vi "Filterwheel.vi"(5 "network settings":T2, 7 "Mode":u16(ring)=1 items=["Init", "Update"], 8 "error in":errorcluster, 10 "Filters&shutters old value":T1={"vis+ND3"=FALSE, "IR+ND2"=FALSE, "Shutter Filterwheel"=TRUE, "Lambda Filterwheel 2"=1, "ND filterwheel 2"=1, "Epi Shutter 2"=FALSE} {"ND filterwheel 2" items=["ND0"=4, "ND1"=6, "ND2"=1, "ND3"=3, "ND4"=2]; "Lambda Filterwheel 2" items=["IR"=1, ""=2, "E440sp"=6]}, 11 "Filters&shutters":T1 {"ND filterwheel 2" items=["ND10"=1, "ND20"=2, "ND30"=3, "ND40"=4, "ND INFINITY"=5, "ND0"=6]; "Lambda Filterwheel 2" items=["IR"=1, "ND50"=2, "ND0"=3, "Green"=4, "Blue"=5, "ND0"=6]}) -> (0 "error out":errorcluster, 2 "String description":string, 3 "Filters&shutters Out":T1 {"ND filterwheel 2" items=["ND10"=1, "ND20"=2, "ND30"=3, "ND40"=4, "ND INFINITY"=5, "ND0"=6]; "Lambda Filterwheel 2" items=["IR"=1, "ND50"=2, "ND0"=3, "Green"=4, "Blue"=5, "ND0"=6]}, 4 "ND FW Strings And Values []":cluster{"String":string, "Value":u16}[](array[cluster]), 6 "Lambda FW Strings And Values []":cluster{"String":string, "Value":u16}[](array[cluster]))   [LabVIEW 2009]
panel:
  in  "Case Constant\n(See Context Help) 4":bool
  in  "Case Constant\n(See Context Help) 3":bool
  in  "Case Constant\n(See Context Help) 2":bool
  in  "Case Constant\n(See Context Help)":bool
  out "Lambda Filterwheel 2":u16(ring)=2 items=["IR"=1, ""=2, "E440sp"=6]
  out "ND filterwheel 2":u16(ring)=1 items=["ND0"=4, "ND1"=6, "ND2"=1, "ND3"=3, "ND4"=2]
  out "EpiShutter":bool
  out "Shutter Filterwheel":bool caption="Filterwheel"
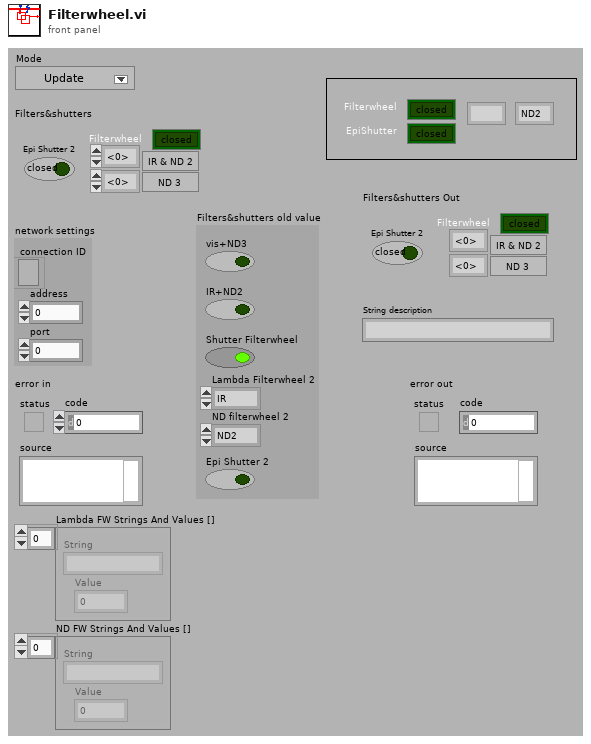
[diagram p1: front panel]
types:
  T1 = cluster{"vis+ND3":bool, "IR+ND2":bool, "Shutter Filterwheel":bool, "Lambda Filterwheel 2":u16, "ND filterwheel 2":u16, "Epi Shutter 2":bool}
  T2 = cluster{"connection ID":refnum<k16>, "address":u32, "port":u16}
  T3 = typedef "LVStringsAndValuesArrayTypeDef.ctl" = cluster{"String":string, "Value":u16}[]
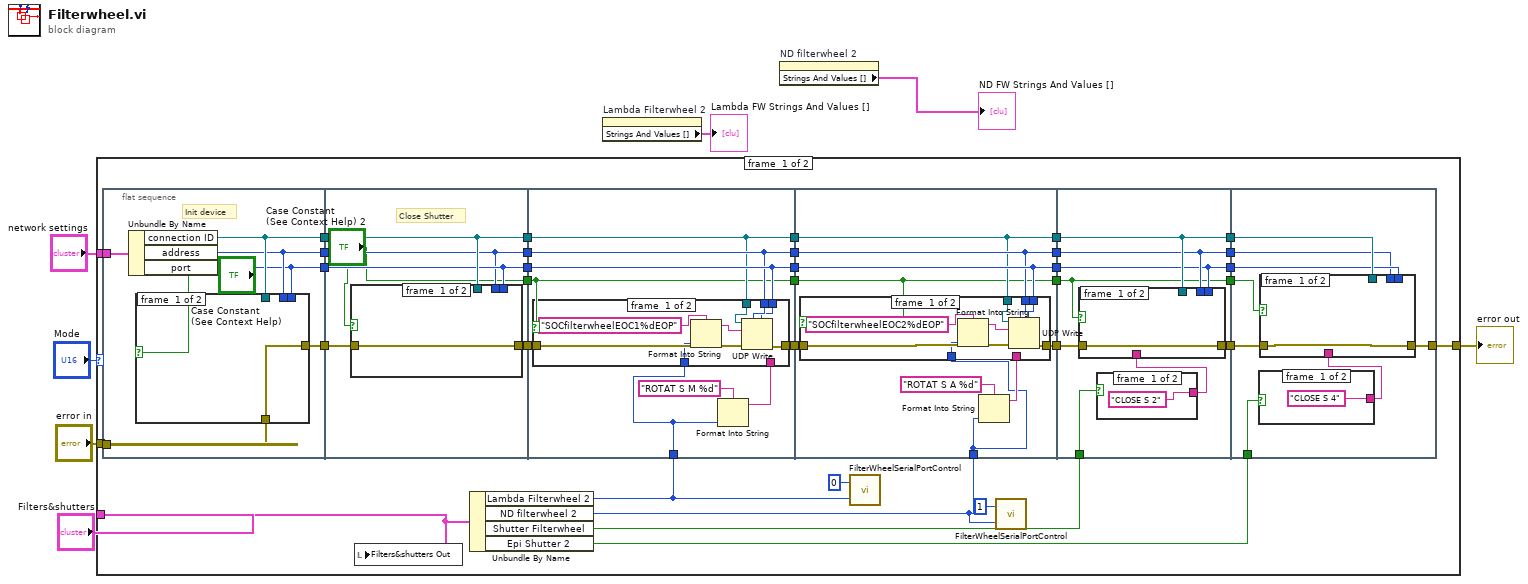
[diagram p0: block diagram]
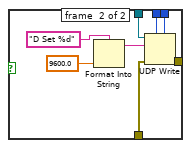
[diagram p2: hidden frame]
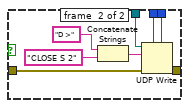
[diagram p3: hidden frame]
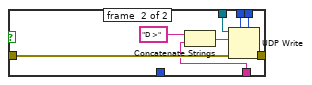
[diagram p4: hidden frame]
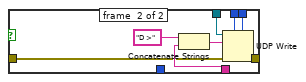
[diagram p5: hidden frame]
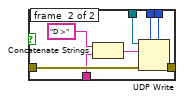
[diagram p6: hidden frame]
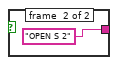
[diagram p7: hidden frame]
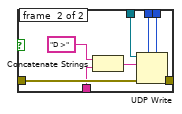
[diagram p8: hidden frame]
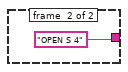
[diagram p9: hidden frame]
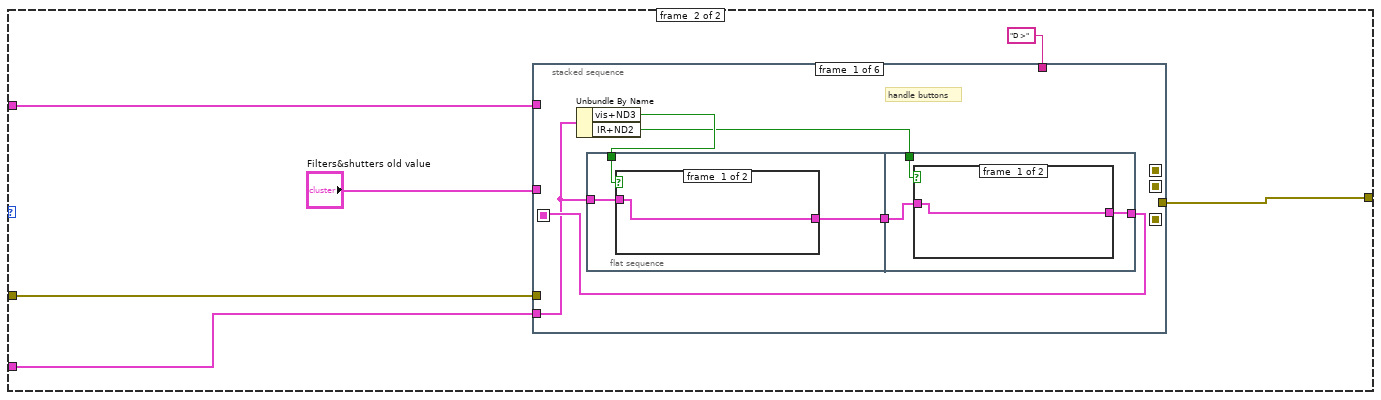
[diagram p10: hidden frame]
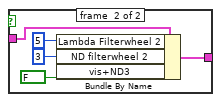
[diagram p11: hidden frame]
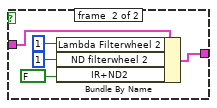
[diagram p12: hidden frame]
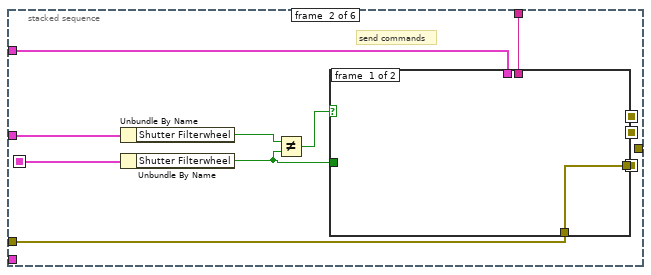
[diagram p13: hidden frame]
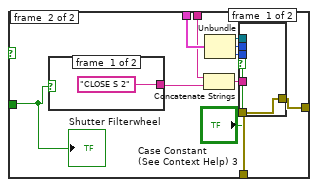
[diagram p14: hidden frame]
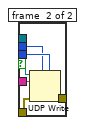
[diagram p15: hidden frame]
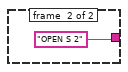
[diagram p16: hidden frame]
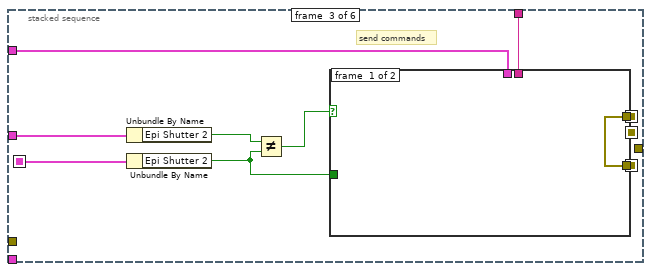
[diagram p17: hidden frame]
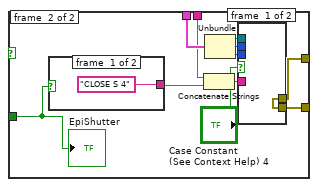
[diagram p18: hidden frame]
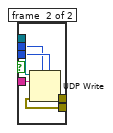
[diagram p19: hidden frame]
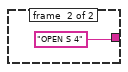
[diagram p20: hidden frame]
diagram:
  n1 = case shown="1, Default" "Mode" {
    tunnel: "network settings" -> [w41 w164]
    tunnel: "error in" -> [w40 w163]
    tunnel: [w39 w162] -> w4
    tunnel: "Filters&shutters" -> [w21 w161]
    frame #0 {
      n2 = flat-sequence {
        tunnel: w41 -> [w48]
        tunnel: w40 -> [w47]
        tunnel: [w46] -> w38
        tunnel: [w45] -> w37
        tunnel: [w44] -> w36
        tunnel: [w43] -> w35
        tunnel: w38 -> [w63]
        tunnel: w37 -> [w61]
        tunnel: w36 -> [w59]
        tunnel: w35 -> [w60]
        tunnel: [w62] -> w34
        tunnel: [w61] -> w33
        tunnel: [w60] -> w32
        tunnel: [w59] -> w31
        tunnel: ["Case Constant\n(See Context Help) 2"] -> w11
        tunnel: w34 -> [w81]
        tunnel: w33 -> [w77]
        tunnel: [w77] -> w29
        tunnel: w32 -> [w79]
        tunnel: [w79] -> w27
        tunnel: w31 -> [w78]
        tunnel: [w78] -> w25
        tunnel: [w80] -> w30
        tunnel: w15 -> [w73]
        tunnel: w11 -> [w74]
        tunnel: [w74] -> w10
        tunnel: w30 -> [w103]
        tunnel: w29 -> [w100]
        tunnel: [w100] -> w28
        tunnel: w27 -> [w102]
        tunnel: [w102] -> w26
        tunnel: w25 -> [w101]
        tunnel: [w101] -> w24
        tunnel: [w104] -> w23
        tunnel: w14 -> [w98]
        tunnel: w10 -> [w99]
        tunnel: [w99] -> w9
        tunnel: w23 -> [w130]
        tunnel: w28 -> [w126]
        tunnel: w26 -> [w124]
        tunnel: w24 -> [w125]
        tunnel: w22 -> [w127]
        tunnel: [w129] -> w20
        tunnel: [w126] -> w19
        tunnel: [w125] -> w18
        tunnel: [w124] -> w17
        tunnel: w9 -> [w123]
        tunnel: [w123] -> w8
        tunnel: [w148] -> w39
        tunnel: w20 -> [w149]
        tunnel: w19 -> [w147]
        tunnel: w18 -> [w145]
        tunnel: w17 -> [w146]
        tunnel: w16 -> [w143]
        tunnel: w8 -> [w142]
        frame #0 {
          # "Init device"
          n3 = Unbundle By Name(w48) -> ("connection ID"=w45:refnum<k16>, "address"=w44:u32, "port"=w43:u16)
          n4 = case shown="True" "Case Constant\n(See Context Help)" {
            tunnel: w47 -> [w49 w54]
            tunnel: [w49 w53] -> w46
            tunnel: w45 -> [_ w52]
            tunnel: w44 -> [_ w51]
            tunnel: w43 -> [_ w50]
            frame #0 {
            }
            frame #1 {
              n5 = Format Into String(format string="D Set %d", 9600.0 ("input 1")) -> (resulting string=w57:string)  [unwired: 2 in, 1 out]
              n6 = UDP Write(address=w51, port or service name=w50, connection ID=w52, data in=w57, 8:w54) -> (error out=w53:errorcluster)  [unwired: 1 in, 1 out]
            }
          }
        }
        frame #1 {
          # "Close Shutter"
          n7 = case shown="True" "Case Constant\n(See Context Help) 2" {
            tunnel: w63 -> [w64 w69]
            tunnel: [w64 w68] -> w62
            tunnel: w61 -> [_ w67]
            tunnel: w60 -> [_ w66]
            tunnel: w59 -> [_ w65]
            frame #0 {
            }
            frame #1 {
              n8 = Concatenate Strings("D >" ("string"), "CLOSE S 2") -> (w70:string)
              n9 = UDP Write(address=w65, port or service name=w66, connection ID=w67, data in=w70, 8:w69) -> (error out=w68:errorcluster)  [unwired: 1 in, 1 out]
            }
          }
        }
        frame #2 {
          n10 = Format Into String(format string="ROTAT S M %d", w73) -> (resulting string=w75:string)  [unwired: 2 in, 1 out]
          n11 = case shown="True" w74 {
            tunnel: w81 -> [w86 w95]
            tunnel: [w85 w94] -> w80
            tunnel: w79 -> [w88 w93]
            tunnel: w78 -> [w89 w92]
            tunnel: w77 -> [w87 w91]
            tunnel: w75 -> [_ w90]
            tunnel: w73 -> [w83 _]
            frame #0 {
              n12 = Format Into String(format string="SOCfilterwheelEOC1%dEOP" ("initial string"), w83) -> (resulting string=w84:string)  [unwired: 2 in, 1 out]
              n13 = UDP Write(address=w89, port or service name=w88, connection ID=w87, data in=w84, 8:w86) -> (error out=w85:errorcluster)  [unwired: 1 in, 1 out]
            }
            frame #1 {
              n14 = Concatenate Strings("D >" ("string"), w90) -> (w96:string)
              n15 = UDP Write(address=w92, port or service name=w93, connection ID=w91, data in=w96, 8:w95) -> (error out=w94:errorcluster)  [unwired: 1 in, 1 out]
            }
          }
        }
        frame #3 {
          n16 = Format Into String(format string="ROTAT S A %d", w98) -> (resulting string=w106:string)  [unwired: 2 in, 1 out]
          n17 = case shown="True" w99 {
            tunnel: w106 -> [_ w122]
            tunnel: [w112 w119] -> w104
            tunnel: w103 -> [w113 w118]
            tunnel: w102 -> [w108 w117]
            tunnel: w101 -> [w109 w116]
            tunnel: w100 -> [w110 w115]
            tunnel: w98 -> [w111 _]
            frame #0 {
              n18 = Format Into String(format string="SOCfilterwheelEOC2%dEOP" ("initial string"), w111) -> (resulting string=w114:string)  [unwired: 2 in, 1 out]
              n19 = UDP Write(address=w109, port or service name=w108, connection ID=w110, data in=w114, 8:w113) -> (error out=w112:errorcluster)  [unwired: 1 in, 1 out]
            }
            frame #1 {
              n20 = Concatenate Strings("D >" ("string"), w122) -> (w121:string)
              n21 = UDP Write(address=w116, port or service name=w117, connection ID=w115, data in=w121, 8:w118) -> (error out=w119:errorcluster)  [unwired: 1 in, 1 out]
            }
          }
        }
        frame #4 {
          n22 = case shown="True" w127 {
            tunnel: ["CLOSE S 2" "OPEN S 2"] -> w128
            frame #0 {
            }
            frame #1 {
            }
          }
          n23 = case shown="True" w123 {
            tunnel: w130 -> [w131 w137]
            tunnel: [w131 w136] -> w129
            tunnel: w128 -> [_ w135]
            tunnel: w126 -> [_ w134]
            tunnel: w125 -> [_ w133]
            tunnel: w124 -> [_ w132]
            frame #0 {
            }
            frame #1 {
              n24 = Concatenate Strings("D >" ("string"), w135) -> (w139:string)
              n25 = UDP Write(address=w133, port or service name=w132, connection ID=w134, data in=w139, 8:w137) -> (error out=w136:errorcluster)  [unwired: 1 in, 1 out]
            }
          }
        }
        frame #5 {
          n26 = case shown="True" w143 {
            tunnel: ["CLOSE S 4" "OPEN S 4"] -> w144
            frame #0 {
            }
            frame #1 {
            }
          }
          n27 = case shown="True" w142 {
            tunnel: w149 -> [w150 w156]
            tunnel: [w150 w155] -> w148
            tunnel: w147 -> [_ w154]
            tunnel: w146 -> [_ w153]
            tunnel: w145 -> [_ w152]
            tunnel: w144 -> [_ w151]
            frame #0 {
            }
            frame #1 {
              n28 = Concatenate Strings("D >" ("string"), w151) -> (w157:string)
              n29 = UDP Write(address=w152, port or service name=w153, connection ID=w154, data in=w157, 8:w156) -> (error out=w155:errorcluster)  [unwired: 1 in, 1 out]
            }
          }
        }
      }
      n30 = local write "Filters&shutters Out"(w21) -> ()
      n31 = Unbundle By Name(w21) -> ("Lambda Filterwheel 2"=w15:u16, "ND filterwheel 2"=w14:u16, "Shutter Filterwheel"=w22:bool, "Epi Shutter 2"=w16:bool)
      n32 = call "FilterWheelSerialPortControl.vi"("position"=w15, "channel"=u8 0) -> ()  [unwired: 1 out]
      n33 = call "FilterWheelSerialPortControl.vi"("position"=w14, "channel"=u8 1) -> ()  [unwired: 1 out]
    }
    frame #1 {
      n34 = stacked-sequence {
        seq-local: [_ w195 _ _ _ _] -> [_ _ w225 _ _ _]
        seq-local: [_ _ w224 _ _ _] -> [_ _ _ w254 w275 _]
        seq-local: [_ _ _ _ w274 _] -> [_ _ _ _ _ w294]
        seq-local: [w168 _ _ _ _ _] -> [_ w192 w221 w251 w271 w293]
        tunnel: w164 -> [_ w198 w228 w257 w278 _]
        tunnel: "D >" ("string") -> [_ w197 w227 w256 w277 _]
        tunnel: w163 -> [_ w190 _ _ _ _]
        tunnel: [_ _ _ _ _ w294] -> w162
        tunnel: "Filters&shutters old value" -> [_ w194 w223 w253 w273 _]
        tunnel: w161 -> [w167 _ _ _ _ _]
        frame #0 {
          # "handle buttons"
          n35 = Unbundle By Name(w167) -> ("vis+ND3"=w170:bool, "IR+ND2"=w169:bool)
          n36 = flat-sequence {
            tunnel: w167 -> [w174]
            tunnel: [w173] -> w171
            tunnel: w170 -> [w172]
            tunnel: w171 -> [w183]
            tunnel: w169 -> [w182]
            tunnel: [w181] -> w168
            frame #0 {
              n37 = case shown="True" w172 {
                tunnel: w174 -> [w175 w180]
                tunnel: [w175 w176] -> w173
                frame #0 {
                }
                frame #1 {
                  n38 = Bundle By Name(cluster=w180, "Lambda Filterwheel 2"=u16 5, "ND filterwheel 2"=u16 3, "vis+ND3"=FALSE) -> (w176:T1)
                }
              }
            }
            frame #1 {
              n39 = case shown="True" w182 {
                tunnel: w183 -> [w184 w189]
                tunnel: [w184 w185] -> w181
                frame #0 {
                }
                frame #1 {
                  n40 = Bundle By Name(cluster=w189, "Lambda Filterwheel 2"=u16 1, "ND filterwheel 2"=u16 1, "IR+ND2"=FALSE) -> (w185:T1)
                }
              }
            }
          }
        }
        frame #1 {
          # "send commands"
          n41 = Unbundle By Name(w194) -> ("Shutter Filterwheel"=w193:bool)
          n42 = Unbundle By Name(w192) -> ("Shutter Filterwheel"=w191:bool)
          n43 = Not Equal?(x=w193, y=w191) -> (x != y?=w196:bool)
          n44 = case shown="True" w196 {
            tunnel: w198 -> [_ w205]
            tunnel: w197 -> [_ w204]
            tunnel: w190 -> [w199 w203]
            tunnel: [w199 w202] -> w195
            tunnel: w191 -> [_ w201]
            frame #0 {
            }
            frame #1 {
              n45 = case shown="False" w201 {
                tunnel: ["CLOSE S 2" "OPEN S 2"] -> w206
                frame #0 {
                }
                frame #1 {
                }
              }
              n46 = Concatenate Strings(w204, w206) -> (w210:string)
              n47 = Unbundle(w205) -> ("connection ID"=w209:refnum<k16>, "address"=w207:u32, "port"=w208:u16)
              n48 = case shown="True" "Case Constant\n(See Context Help) 3" {
                tunnel: w210 -> [_ w217]
                tunnel: w209 -> [_ w216]
                tunnel: w208 -> [_ w215]
                tunnel: w207 -> [_ w214]
                tunnel: w203 -> [w211 w213]
                tunnel: [w211 w212] -> w202
                frame #0 {
                }
                frame #1 {
                  n49 = UDP Write(address=w214, port or service name=w215, connection ID=w216, data in=w217, 8:w213) -> (error out=w212:errorcluster)  [unwired: 1 in, 1 out]
                }
              }
              "Shutter Filterwheel" <- w201
            }
          }
        }
        frame #2 {
          # "send commands"
          n50 = Unbundle By Name(w223) -> ("Epi Shutter 2"=w222:bool)
          n51 = Unbundle By Name(w221) -> ("Epi Shutter 2"=w220:bool)
          n52 = Not Equal?(x=w222, y=w220) -> (x != y?=w226:bool)
          n53 = case shown="True" w226 {
            tunnel: w228 -> [_ w235]
            tunnel: w227 -> [_ w234]
            tunnel: w225 -> [w229 w233]
            tunnel: [w229 w232] -> w224
            tunnel: w220 -> [_ w231]
            frame #0 {
            }
            frame #1 {
              n54 = case shown="True" w231 {
                tunnel: ["CLOSE S 4" "OPEN S 4"] -> w236
                frame #0 {
                }
                frame #1 {
                }
              }
              n55 = Concatenate Strings(w234, w236) -> (w240:string)
              n56 = Unbundle(w235) -> ("connection ID"=w239:refnum<k16>, "address"=w237:u32, "port"=w238:u16)
              n57 = case shown="True" "Case Constant\n(See Context Help) 4" {
                tunnel: w240 -> [_ w247]
                tunnel: w239 -> [_ w246]
                tunnel: w238 -> [_ w245]
                tunnel: w237 -> [_ w244]
                tunnel: w233 -> [w241 w243]
                tunnel: [w241 w242] -> w232
                frame #0 {
                }
                frame #1 {
                  n58 = UDP Write(address=w244, port or service name=w245, connection ID=w246, data in=w247, 8:w243) -> (error out=w242:errorcluster)  [unwired: 1 in, 1 out]
                }
              }
              "EpiShutter" <- w231
            }
          }
        }
        frame #3 {
          # "send commands"
          n59 = Unbundle By Name(w253) -> ("Lambda Filterwheel 2"=w252:u16)
          n60 = Unbundle By Name(w251) -> ("Lambda Filterwheel 2"=w250:u16)
          n61 = Not Equal?(x=w252, y=w250) -> (x != y?=w255:bool)
          n62 = case shown="True" w255 {
            tunnel: w257 -> [_ w266]
            tunnel: w256 -> [_ w265]
            tunnel: w254 -> [_ w262]
            tunnel: w250 -> [_ w260]
            frame #0 {
            }
            frame #1 {
              n63 = call "FilterWheelSerialPortControl.vi"("position"=w260, "channel"=u8 0) -> ()  [unwired: 1 out]
              n64 = Format Into String(format string="ROTAT S M %d", w260) -> (resulting string=w263:string)  [unwired: 2 in, 1 out]
              n65 = Unbundle(w266) -> ("connection ID"=w269:refnum<k16>, "address"=w267:u32, "port"=w268:u16)
              n66 = Concatenate Strings(w265, w263) -> ()  [unwired: 1 out]
              n67 = Format Into String(format string="SOCfilterwheelEOC0,%dEOP" ("initial string"), w260) -> (resulting string=w259:string)  [unwired: 2 in, 1 out]
              n68 = UDP Write(address=w267, port or service name=w268, connection ID=w269, data in=w259, 8:w262) -> ()  [unwired: 1 in, 2 out]
              "Lambda Filterwheel 2" <- w260
            }
          }
        }
        frame #4 {
          # "send commands"
          n69 = Unbundle By Name(w273) -> ("ND filterwheel 2"=w272:u16)
          n70 = Unbundle By Name(w271) -> ("ND filterwheel 2"=w270:u16)
          n71 = Not Equal?(x=w272, y=w270) -> (x != y?=w276:bool)
          n72 = case shown="True" w276 {
            tunnel: w278 -> [_ w289]
            tunnel: w277 -> [_ w288]
            tunnel: w275 -> [w279 w285]
            tunnel: [w279 w284] -> w274
            tunnel: w270 -> [_ w282]
            frame #0 {
            }
            frame #1 {
              n73 = call "FilterWheelSerialPortControl.vi"("position"=w282, "channel"=u8 1) -> ()  [unwired: 1 out]
              n74 = Format Into String(format string="ROTAT S A %d", w282) -> (resulting string=w286:string)  [unwired: 2 in, 1 out]
              n75 = Unbundle(w289) -> ("connection ID"=w292:refnum<k16>, "address"=w290:u32, "port"=w291:u16)
              n76 = Concatenate Strings(w288, w286) -> ()  [unwired: 1 out]
              n77 = Format Into String(format string="SOCfilterwheelEOC1,%dEOP" ("initial string"), w282) -> (resulting string=w281:string)  [unwired: 2 in, 1 out]
              n78 = UDP Write(address=w290, port or service name=w291, connection ID=w292, data in=w281, 8:w285) -> (error out=w284:errorcluster)  [unwired: 1 in, 1 out]
              "ND filterwheel 2" <- w282
            }
          }
        }
        frame #5 {
          # "create string"
          n79 = flat-sequence {
            tunnel: w293 -> [w295]
            frame #0 {
              "Filters&shutters Out" <- w295
            }
            frame #1 {
              n80 = property on="Lambda Filterwheel 2" class="Ring (strict)"() -> ("Ring Text.Text"=w298:string)  [unwired: 2 in, 2 out]
              n81 = property on="ND filterwheel 2" class="Ring (strict)"() -> ("Ring Text.Text"=w299:string)  [unwired: 2 in, 2 out]
              n82 = Concatenate Strings("_" ("string"), w298, w299) -> (→"String description":string)
            }
          }
        }
      }
    }
  }
  "error out" <- w4
  n83 = property on="Lambda Filterwheel 2" class="Ring (strict)"() -> ("Strings And Values []"=→"Lambda FW Strings And Values []":T3)  [unwired: 2 in, 2 out]
  n84 = property on="ND filterwheel 2" class="Ring (strict)"() -> ("Strings And Values []"=→"ND FW Strings And Values []":T3)  [unwired: 2 in, 2 out]
